vi "Add Points to XY Array.vi"(9 "Parameter":dbl, 10 "Values":dbl[](array[numeric]), 11 "Array in":cluster{"X":dbl[], "Y":dbl[]}[](array[cluster])) -> (3 "Array out":cluster{"X":dbl[], "Y":dbl[]}[](array[cluster]))   [LabVIEW 2014, in "MassSpectrumExtractor.lvclass"]
uses:
  MassSpectrumExtractor.lvclass
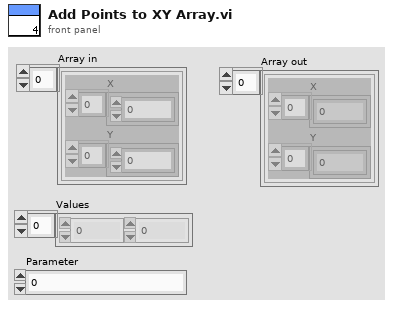
[diagram p1: front panel]
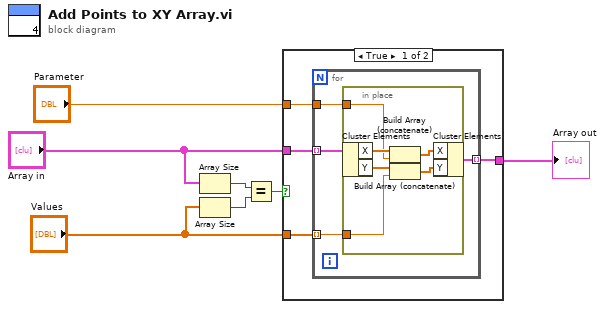
[diagram p0: block diagram]
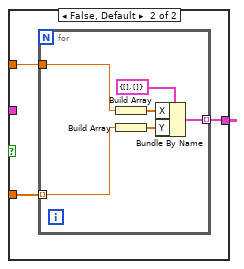
[diagram p2: hidden frame]
diagram:
  n1 = Array Size(array="Array in") -> (size(s)=w1:i32)
  n2 = Array Size(array="Values") -> (size(s)=w2:i32)
  n3 = Equal?(x=w1, y=w2) -> (x = y?=w3:bool)
  n4 = case shown="True" w3 {
    tunnel: "Values" -> [w10 w24]
    tunnel: "Array in" -> [w11 _]
    tunnel: "Parameter" -> [w9 w23]
    tunnel: [w8 w22] -> w7
    frame True {
      n5 = for {
        tunnel: w11 -> [w15] mode=indexing
        tunnel: w10 -> [w13] mode=indexing
        tunnel: w9 -> [w14]
        tunnel: [w12] -> w8 mode=indexing
        n6 = in-place {
          in-place-border: w14 -> [w20]
          in-place-border: w13 -> [w18]
          n7 = in-place-cluster #1(w15) -> ("X"=w21:dbl[], "Y"=w19:dbl[])
          n8 = Build Array (concatenate)(w21, w20) -> (w17:dbl[])
          n9 = Build Array (concatenate)(w19, w18) -> (w16:dbl[])
          n10 = in-place-cluster #1("X"=w17, "Y"=w16) -> (w12:cluster{"X":dbl[], "Y":dbl[]})
        }
      }
    }
    frame False, Default {
      n11 = for {
        tunnel: w24 -> [w29] mode=indexing
        tunnel: w23 -> [w30]
        tunnel: [w27] -> w22 mode=indexing
        n12 = Build Array(w30) -> (w26:dbl[])
        n13 = Build Array(w29) -> (w28:dbl[])
        n14 = Bundle By Name(cluster=cluster{"X":dbl[], "Y":dbl[]} {"X"=[], "Y"=[]}, "X"=w26, "Y"=w28) -> (w27:cluster{"X":dbl[], "Y":dbl[]})
      }
    }
  }
  "Array out" <- w7
